vi "ReadBusDataFromFile.vi"(8 "ErrorArray In":errorcluster[](array[cluster]), 11 "TestFileRef In":T11) -> (0 "ErrorArray Out":errorcluster[](array[cluster]), 1 "BusData":T1[](array[typedef]) {"clConfigOptions"."PHUNIT" max=16777216 step=1 format="%08d"; "clConfigOptions"."IDCODE" format="%02x"; "clConfigOptions"."TIME_BASE" max=16777216 step=1 format="%08d"; "ImpairReportArray"."Synx" format="%#_4g"; "EvtReportArray"."Synx" format="%#_4g"; "EvtConfig"."Reporting Rate" items=["10 FPS"=10, "12 FPS"=12, "15 FPS"=15, "20 FPS"=20, "25 FPS"=25, "30 FPS"=30, "50 FPS"=50, "60 FPS"=60]; "EvtConfig"."Nominal Frequency" items=["50 Hz"=50, "60 Hz"=60]}, 3 "refnum out":T11)   [LabVIEW 2014, in "Framework.lvlib"]
uses:
  Framework.lvlib
  <vilib>/Utility/config.llb/Config Data RefNum.ctl
  Bus_class/Public/TypeDefs/clBusData.ctl
  FrontPanel/TypeDefs/clEventConfig.ctl
  Modules/PmuImpairPlugins/PmuImpairPluginBase_class/TypeDefs/clImpairConfig.ctl
  Modules/EventPlugins/EventPluginBaseClass/TypeDefs/clEvtReportArray.ctl
  Modules/EventPlugins/EventPluginBaseClass/TypeDefs/clEvtReport.ctl
  Modules/EventPlugins/EventPluginBaseClass/TypeDefs/dblEvtSignalArray.ctl
  Modules/NetworkImpairmentModule/PublicAPI/Arguments/Broadcasts/dblNetworkTime.ctl
  Modules/NetworkImpairmentModule/PublicAPI/Arguments/Broadcasts/dblPktLoss.ctl
  Modules/FlagImpairModule/PublicAPI/Arguments/Broadcasts/ui32FlagImpairmentArray.ctl
  Modules/OutputToFilePlugins/OutputToFileBasePlugin/Typedefs/PmuCfgOpt.ctl
  Bus_class/Public/TypeDefs/clBusSaveData.ctl
  <userlib>/NIST/NISTErrorLib/NISTErrorLib.lvlib
  <vilib>/Utility/config.llb/NI_LVConfig.lvlib
  Bus_class/Bus.lvclass
  Modules/EventPlugins/EventPluginBaseClass/EventPluginBaseClass.lvclass
  Modules/NetworkImpairmentModule/NetworkImpairmentModule.lvlib
  Modules/FlagImpairModule/FlagImpairModule.lvlib
  Modules/OutputToFilePlugins/OutputToFileBasePlugin/OutputToFileBasePlugin.lvclass
  Modules/PmuImpairPlugins/PmuImpairPluginBase_class/PmuImpairPluginBase.lvclass
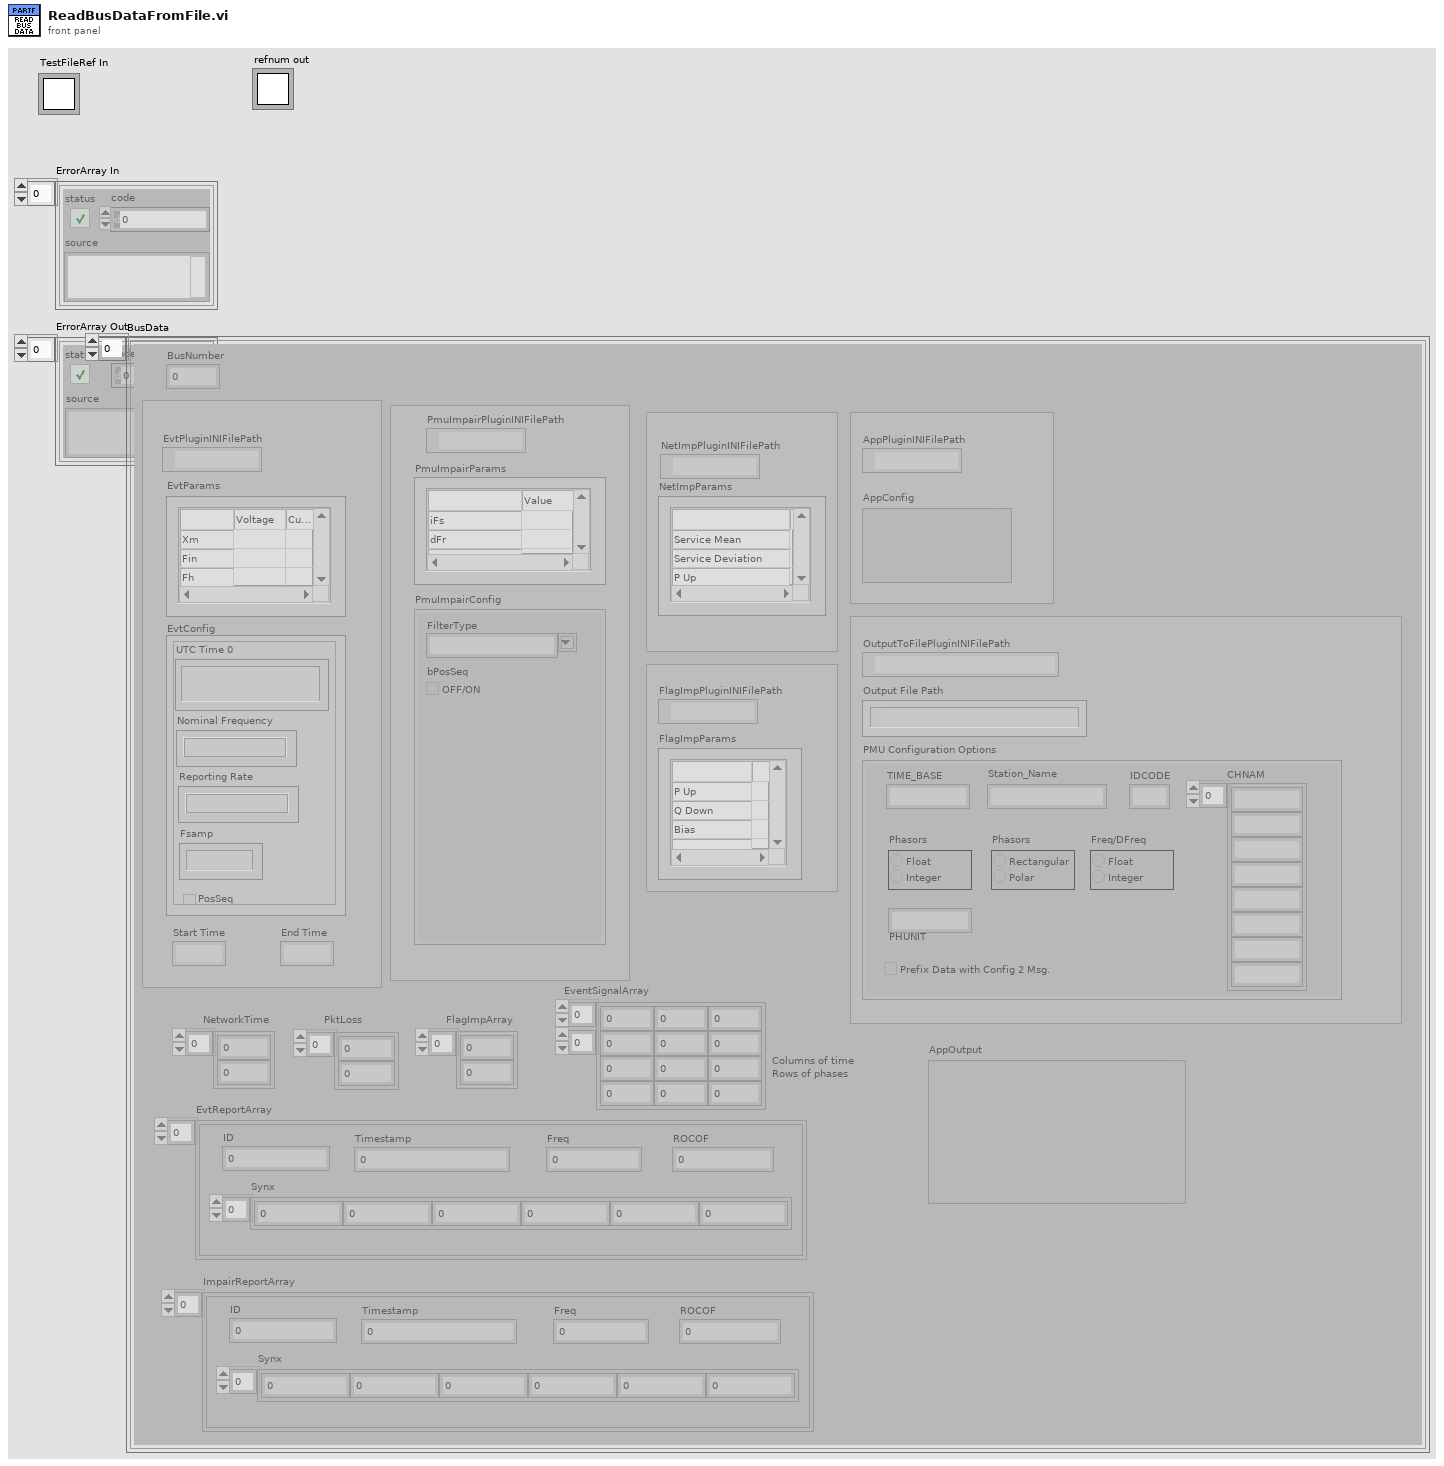
[diagram p1: front panel]
types:
  T1 = typedef "Bus_class.lvlib/Bus.lvclass/clBusData.ctl" = cluster{"BusNumber":u8, "EvtPluginINIFilePath":path, "EvtParams":string[][], "EvtConfig":T2, "Start Time":dbl, "End Time":dbl, "PmuImpairPluginINIFilePath":path, "PmuImpairParams ":string[][], "PmuImpairConfig":T3, "NetImpPluginINIFilePath":path, "NetImpParams":string[][], "FlagImpPluginINIFilePath":path, "FlagImpParams":string[][], "EvtReportArray":T4, "EventSignalArray":T6, "ImpairReportArray":T4, "NetworkTime":T7, "PktLoss":T8, "FlagImpArray":T9, "OutputToFilePluginINIFilePath":path, "Output File Path":path, "clConfigOptions":T10, "AppPluginINIFilePath":path, "AppConfig":variant, "AppOutput":variant}
  T2 = typedef "Framework.lvlib/clEventConfig.ctl" = cluster{"UTC Time 0":timestamp, "Nominal Frequency":u16, "Reporting Rate":u16, "Fsamp":u32, "PosSeq":bool}
  T3 = typedef "PmuImpairPlugins.lvlib/PmuImpairPluginBase.lvclass/clImpairConfig.ctl" = cluster{"FilterType":string, "bPosSeq":bool}
  T4 = typedef "EventPlugins.lvlib/EventPluginBaseClass.lvclass/clEvtReportArray.ctl" = T5[]
  T5 = typedef "EventPlugins.lvlib/EventPluginBaseClass.lvclass/clEvtReport.ctl" = cluster{"Timestamp":dbl, "Synx":cdb[], "Freq":dbl, "ROCOF":dbl, "ID":i16}
  T6 = typedef "EventPlugins.lvlib/EventPluginBaseClass.lvclass/dblEvtSignalArray.ctl" = dbl[][]
  T7 = typedef "NetworkImpairmentModule.lvlib/dblNetworkTime.ctl" = dbl[]
  T8 = typedef "NetworkImpairmentModule.lvlib/dblPktLoss.ctl" = dbl[]
  T9 = typedef "FlagImpairModule.lvlib/ui32FlagImpairmentArray.ctl" = u32[]
  T10 = typedef "OutputToFilePlugins.lvlib/OutputToFileBasePlugin.lvclass/PmuCfgOpt.ctl" = cluster{"TIME_BASE":u64, "STN":string, "IDCODE":u16, "rdoPolRect":enum32{"Rectangular", "Polar"}, "rdoFloatInt":enum32{"Float", "Integer"}, "PHUNIT":u64, "rdoFreqDfreq":enum32{"Float", "Integer"}, "CHNAM":string[], "chkCfg2Prefix":bool}
  T11 = typedef "NI_LVConfig.lvlib/Config Data RefNum.ctl" = refnum<k1>
  T12 = typedef "Bus_class.lvlib/Bus.lvclass/clBusSaveData.ctl" = cluster{"EvtPluginINIFilePath":path, "EvtParams":string[][], "EvtConfig":T2, "BusNumber":u8, "Start Time":dbl, "End Time":dbl, "PmuImpairPluginINIFilePath":path, "PmuImpairParams ":string[][], "PmuImpairConfig":T3, "NetImpPluginINIFilePath":path, "NetImpParams":string[][], "FlagImpPluginINIFilePath":path, "FlagImpParams":string[][]}
  T13 = typedef "Framework.lvlib/clFrameworkData.ctl" = cluster{"EvtINIFilePaths":path[], "BusClassInstances":refnum<class "Bus.lvclass">[], "PmuImpairINIFilePaths":path[], "FlagImpairINIFilePaths":path[], "NetImpairINIFilePaths":path[], "OutputToFileINIFilePaths":path[], "AppINIFilePaths":path[], "AppModuleID":i32, "OutputToFileID":i32}
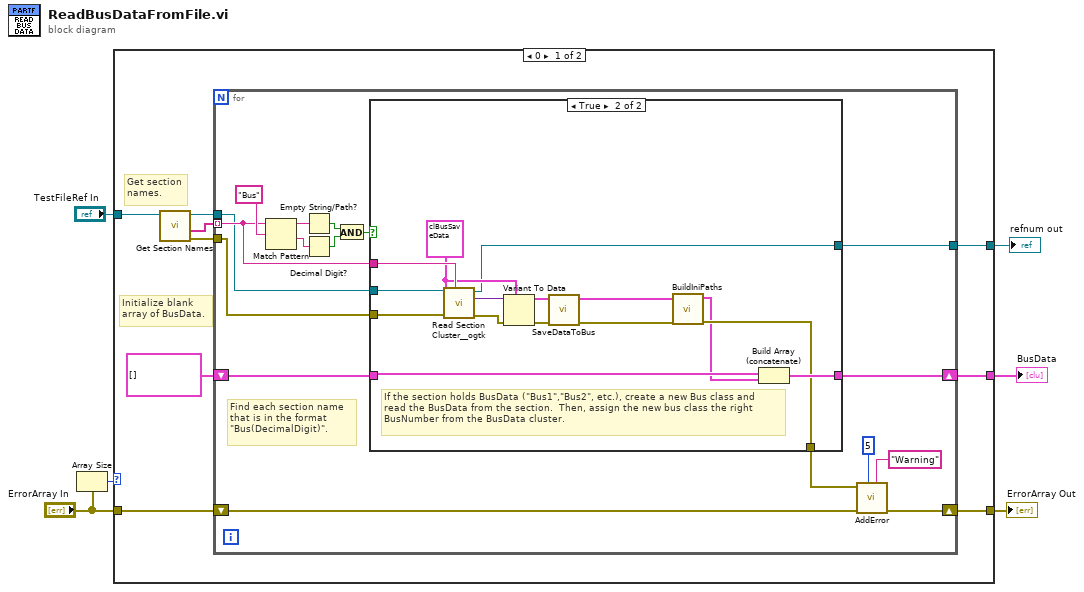
[diagram p0: block diagram]
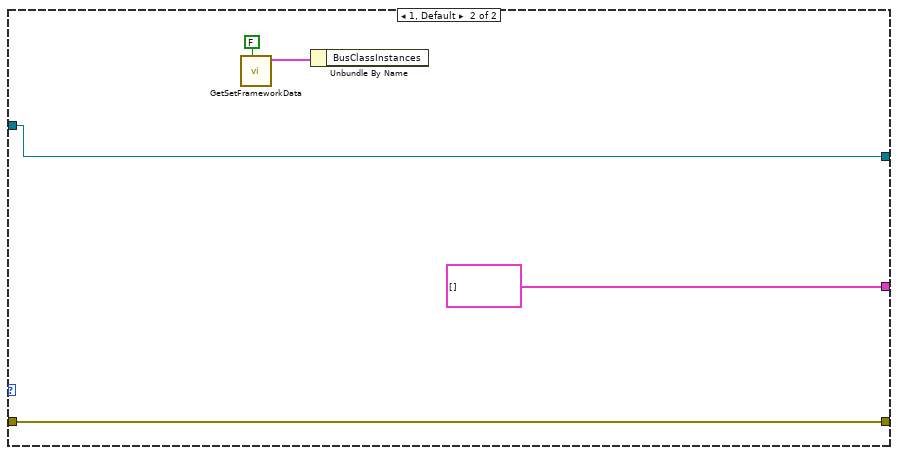
[diagram p3: hidden frame]
diagram:
  n1 = Array Size(array="ErrorArray In") -> (size(s)=w6:i32)
  n2 = case shown="0" w6 {
    tunnel: "ErrorArray In" -> [w15 w55]
    tunnel: [w10 w55] -> w4
    tunnel: "TestFileRef In" -> [w11 w52]
    tunnel: [w8 T1[] []] -> w2
    tunnel: [w7 w52] -> w1
    frame 0 {
      # "Get section\nnames."
      # "Initialize blank\narray of BusData."
      n3 = call <vilib>:"Get Section Names.vi"("refnum"=w11) -> ("error out"=w14:errorcluster, "section names"=w13:string[], "refnum out"=w12:T11)  [unwired: 8 in]
      n4 = for {
        tunnel: w13 -> [w22] mode=indexing
        tunnel: w12 -> [w20]
        shift-right: [w30] -> w10
        shift-left: w15 -> [w31]
        tunnel: w14 -> [w19]
        shift-right: [w17] -> w8
        shift-left: T1[] [] -> [w18]
        tunnel: [w16] -> w7
        # "Find each section name\nthat is in the format\n\"Bus(DecimalDigit)\"."
        n5 = Match Pattern(string=w22, regular expression="Bus") -> (before substring=w26:string, after substring=w25:string)  [unwired: 1 in, 2 out]
        n6 = Empty String/Path?(string/path=w26) -> (empty?=w24:bool)
        n7 = Decimal Digit?(1:w25) -> (0:w23:bool)
        n8 = And(x=w24, y=w23) -> (x .and. y?=w21:bool)
        n9 = case shown="True" w21 {
          tunnel: [w33 w41] -> w28
          tunnel: w22 -> [_ w49]
          tunnel: w20 -> [w34 w50]
          tunnel: w19 -> [w33 w48]
          tunnel: w18 -> [w35 w44]
          tunnel: [w35 w43] -> w17
          tunnel: [w34 w42] -> w16
          frame False {
          }
          frame True {
            w46 = T12 {"EvtPluginINIFilePath"=path "", "EvtParams"=[], "EvtConfig"={"UTC Time 0"=timestamp(0 s since 1904-01-01), "Nominal Frequency"=60, "Reporting Rate"=60, "Fsamp"=960, "PosSeq"=FALSE}, "BusNumber"=0, "Start Time"=0.0, "End Time"=0.0, "PmuImpairPluginINIFilePath"=path "", "PmuImpairParams "=[["960"], ["8.19"], ["164"]], "PmuImpairConfig"={"FilterType"="", "bPosSeq"=TRUE}, "NetImpPluginINIFilePath"=path "", "NetImpParams"=[], "FlagImpPluginINIFilePath"=path "", "FlagImpParams"=[]} ("clEvtData")
            # "If the section holds BusData (\"Bus1\",\"Bus2\", etc.), create a new Bus class and\nread the BusData from the section.  Then, assign the new bus class the right\nBusNumber from the BusData cluster."
            n10 = call <userlib>:"Read Section Cluster__ogtk.vi"("section (optional)"=w49, "error in (no error)"=w48, "Section Formatted Cluster Type"=w46, "refnum"=w50) -> ("error out"=w45:errorcluster, "Section Formatted Cluster"=w47:variant, "dup refnum"=w42:T11)  [unwired: 3 in, 2 out]
            n11 = Variant To Data(error in=w45, type=w46, Variant=w47) -> (data=w38:T12, error out=w39:errorcluster)
            n12 = call "SaveDataToBus.vi"("error in (no error)"=w39, "clBusSaveData"=w38) -> ("error out"=w36:errorcluster, "clBusData"=w37:T1)  [unwired: 8 in]
            n13 = call "BuildIniPaths.vi"("error in (no error)"=w36, "clBusData"=w37) -> ("error out"=w41:errorcluster, "clBusData"=w40:T1)  [unwired: 8 in]
            n14 = Build Array (concatenate)(w44, w40) -> (w43:T1[])
          }
        }
        n15 = call <userlib>:"AddError.vi"("Severity"="Warning" ("String"), "Priority"=u8 5, "ErrorArray"=w31, "error in (no error)"=w28) -> ("ErrorArray"=w30:errorcluster[])  [unwired: 6 in, 1 out]
      }
    }
    frame 1, Default {
      n16 = call "GetSetFrameworkData.vi"("Set (F)"=FALSE ("Set/Get")) -> ("clFrameworkData Out"=w53:T13)  [unwired: 10 in]
      n17 = Unbundle By Name(w53) -> ()  [unwired: 1 out]
    }
  }
  "ErrorArray Out" <- w4
  "refnum out" <- w1
  "BusData" <- w2
